vi "Override Error.vi"(10 "Error":errorcluster, 11 "Ex Event Actor in":refnum<class "Ex Event Actor.lvclass">) -> (3 "Ex Event Actor out":refnum<class "Ex Event Actor.lvclass">)   [LabVIEW 2021, in "Ex Event Actor.lvlib" / "Ex Event Actor.lvclass"]
uses:
  Ex Event Actor.lvclass
  Ex Event Actor.lvclass/Ex Event Actor.ctl
  Actor/Event Actor/Event Actor.lvclass
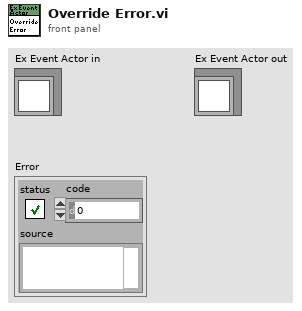
[diagram p1: front panel]
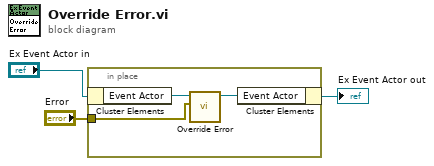
[diagram p0: block diagram]
diagram:
  n1 = in-place {
    in-place-border: "Error" -> [w4]
    n2 = in-place-cluster #1("Ex Event Actor in") -> ("Event Actor"=w6:refnum<class "Event Actor.lvclass">)
    n3 = call-dynamic "Override Error.vi"("Error"=w4, "Override Error in"=w6) -> ("Override Error out"=w5:refnum<class "Event Actor.lvclass">)  [unwired: 9 in]
    n4 = in-place-cluster #1("Event Actor"=w5) -> (→"Ex Event Actor out":refnum<class "Ex Event Actor.lvclass">)
  }
